vi "SET_Show.vi"(8 "error in (no error)":errorcluster, 9 "Show Terminals?":bool, 10 "Show Layer Tab?":bool, 11 "Settings.lvclass in":refnum<class "Settings.lvclass">) -> (0 "error out":errorcluster, 3 "Settings.lvclass out":refnum<class "Settings.lvclass">)   [LabVIEW 2021, in "Settings.lvclass"]
uses:
  <resource>/plugins/NIIconEditor/Class/Settings/Settings.lvclass
  <resource>/plugins/NIIconEditor/Class/Settings/Settings.lvclass/Settings.ctl
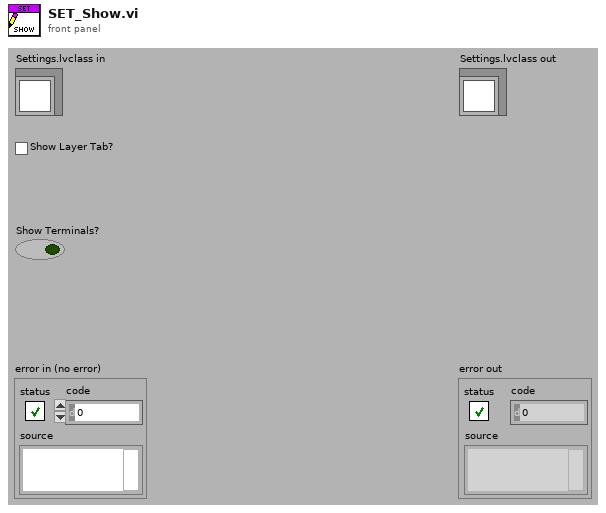
[diagram p1: front panel]
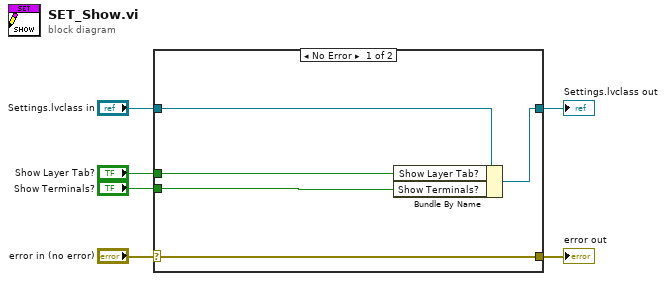
[diagram p0: block diagram]
diagram:
  n1 = case shown="No Error" "error in (no error)" {
    selector: "error in (no error)" -> [w11 w12]
    tunnel: [w11 w12] -> w5
    tunnel: [w9 w13] -> w3
    tunnel: "Settings.lvclass in" -> [w10 w13]
    tunnel: "Show Layer Tab?" -> [w8 _]
    tunnel: "Show Terminals?" -> [w7 _]
    frame No Error {
      n2 = Bundle By Name(cluster=w10, "Show Layer Tab?"=w8, "Show Terminals?"=w7) -> (w9:refnum<class "Settings.lvclass">)
    }
    frame Error {
    }
  }
  "error out" <- w5
  "Settings.lvclass out" <- w3
